vi "KG set cp sp.vi"(8 "Fehler (Eingang, kein Fehler)":errorcluster, 9 "Concentration":dbl, 10 "pump":u32, 11 "VISA-Ressourcenname":refnum<visa-resource-name>) -> (0 "Fehler (Ausgang)":errorcluster, 2 "Kommando gesendet":string, 3 "VISA-Ressourcenname (Ausgang)":refnum<visa-resource-name>)   [LabVIEW 2020, in "Linearisierung v2.lvlib" / "Gasteiler.lvlib" / "HovaCAL_Interface.lvlib" / "KGN.lvlib" / "set.lvlib"]
uses:
  set.lvlib
  KGN.lvlib
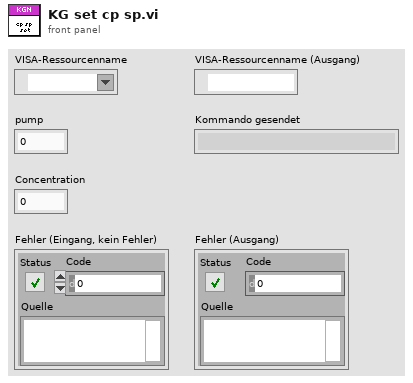
[diagram p1: front panel]
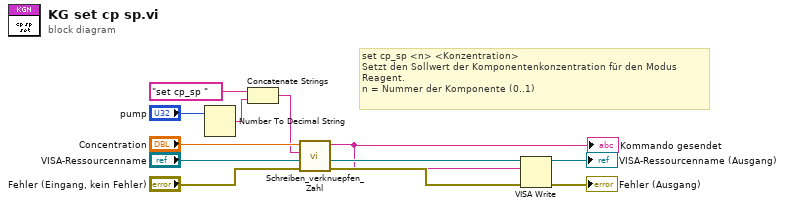
[diagram p0: block diagram]
diagram:
  # "set cp_sp <n> <Konzentration>\nSetzt den Sollwert der Komponentenkonzentration für den Modus\nReagent.\nn = Nummer der Komponente (0..1)"
  n1 = Number To Decimal String(number="pump") -> (decimal integer string=w6:string)  [unwired: 1 in]
  n2 = Concatenate Strings("set cp_sp " ("Schreibpuffer"), w6) -> (w4:string)
  n3 = call "Schreiben_verknuepfen_Zahl.vi"("error in (no error)"="Fehler (Eingang, kein Fehler)", "Order"=w4, "Zahl"="Concentration") -> ("error out"=w2:errorcluster, "Verknüpfter String"=w1:string)  [unwired: 7 in]
  "Kommando gesendet" <- w1
  n4 = VISA Write(VISA resource name="VISA-Ressourcenname", write buffer=w1, error in (no error)=w2) -> (VISA resource name out=→"VISA-Ressourcenname (Ausgang)":refnum<visa-resource-name>, error out=→"Fehler (Ausgang)":errorcluster)  [unwired: 1 out]
